vi "Constrcut.vi"(8 "error in (no error)":errorcluster, 11 "PrintLine":T1) -> (0 "error out":errorcluster, 3 "PrintF out":refnum<class "PrintF.lvclass">)   [LabVIEW 2020, in "UpstreamMsg.lvlib" / "PrintF.lvclass"]
uses:
  PrintF.lvclass
  Msg.ctl
  PrintF.lvclass/PrintF.ctl
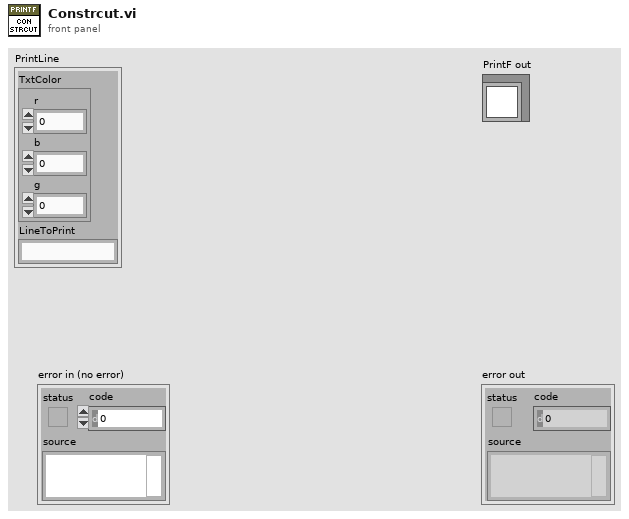
[diagram p1: front panel]
types:
  T1 = typedef "UpstreamMsg.lvlib/PrintF.lvclass/Msg.ctl" = cluster{"TxtColor":cluster{"r":u8, "b":u8, "g":u8}, "LineToPrint":string}
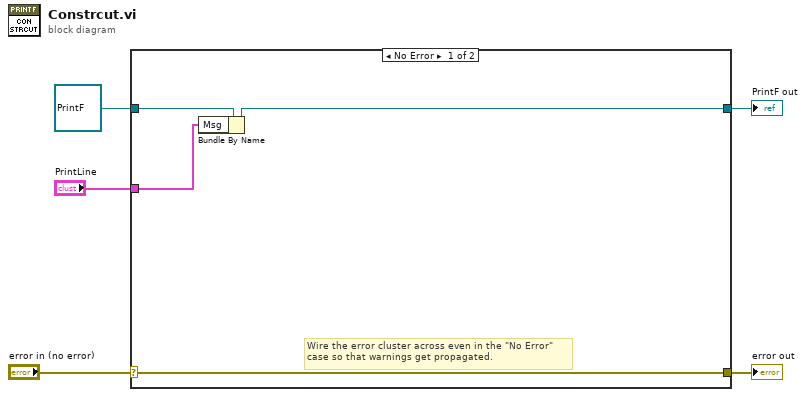
[diagram p0: block diagram]
diagram:
  n1 = case shown="No Error" "error in (no error)" {
    selector: "error in (no error)" -> [w8 w11]
    tunnel: [w8 w11] -> w4
    tunnel: [w7 w10] -> w2
    tunnel: refnum<class "PrintF.lvclass"> refnum ("PrintF in") -> [w9 w10]
    tunnel: "PrintLine" -> [w6 _]
    frame No Error {
      # "Wire the error cluster across even in the \"No Error\"\ncase so that warnings get propagated."
      n2 = Bundle By Name(cluster=w9, "Msg"=w6) -> (w7:refnum<class "PrintF.lvclass">)
    }
    frame Error {
    }
  }
  "error out" <- w4
  "PrintF out" <- w2
